vi "Gui.vi"(0 "reference in":refnum<class "RemoteControl.lvclass">, 5 "error in (no error)":errorcluster) -> (14 "reference out":refnum<class "RemoteControl.lvclass">, 19 "error out":errorcluster)   [LabVIEW 2012, in "RemoteControl.lvclass"]
uses:
  RemoteControl.lvclass
  Command_class/Command.lvclass
panel:
  in  "UndoLastCommand":bool
  in  "Slot2_Off":bool
  in  "Slot2_On":bool
  in  "Slot1_Off":bool
  in  "Slot1_On":bool
  in  "Slot0_Off":bool
  in  "Slot0_On":bool
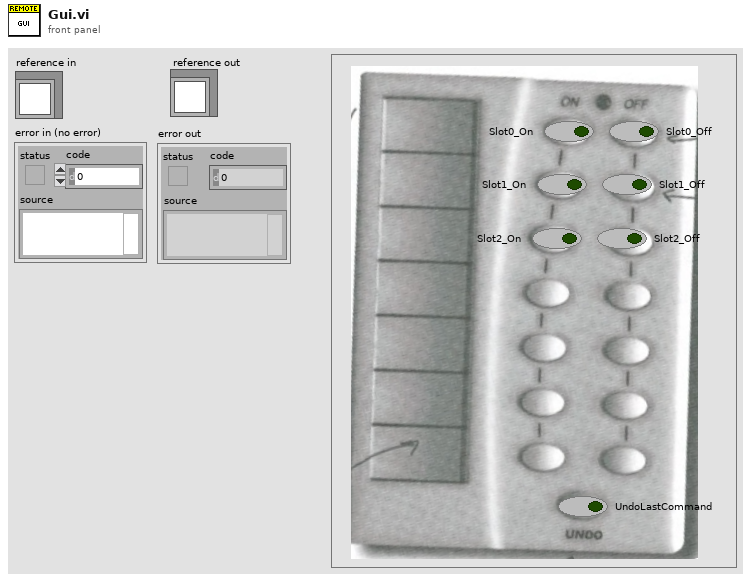
[diagram p1: front panel]
types:
  T1 = cluster{"Event":refnum<event-registration>, "Command":string, "Data":variant, "UndoCommand":refnum<class "Command.lvclass">}
  T2 = typedef "RemoteControl.lvclass/ObjectAttributes.ctl" = cluster{"OnCommands":refnum<class "Command.lvclass">[], "OffCommands":refnum<class "Command.lvclass">[], "UndoCommand":refnum<class "Command.lvclass">}
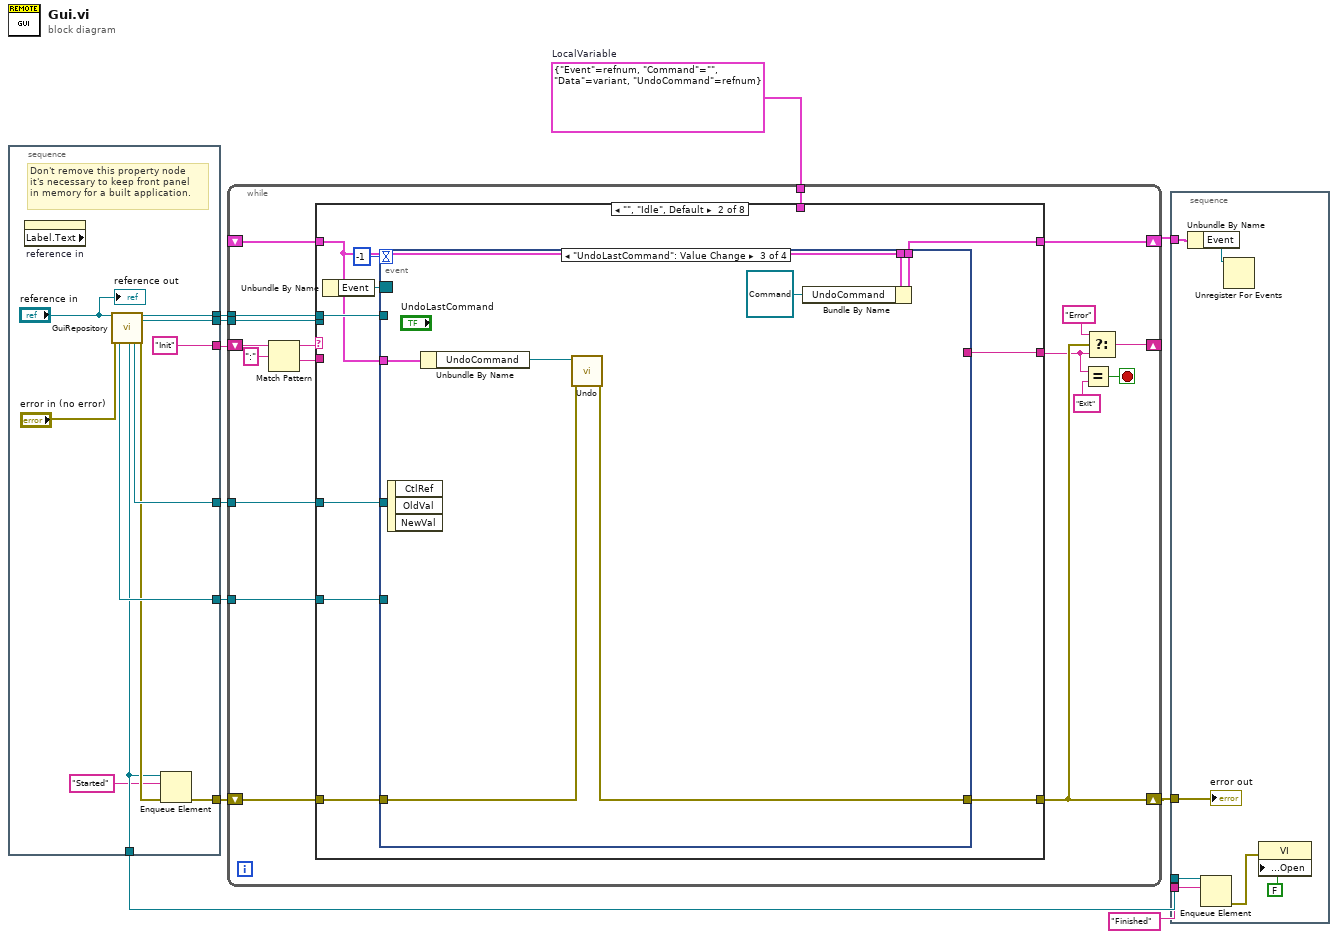
[diagram p0: block diagram]
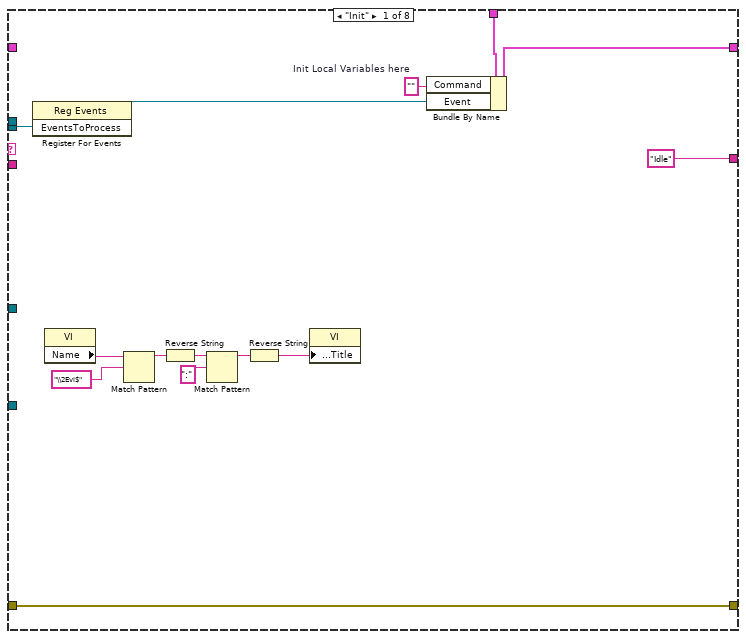
[diagram p2: hidden frame]
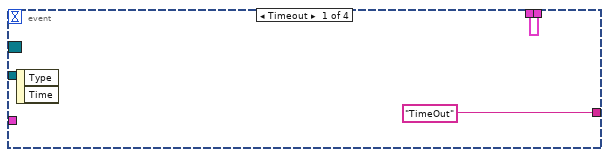
[diagram p3: hidden frame]
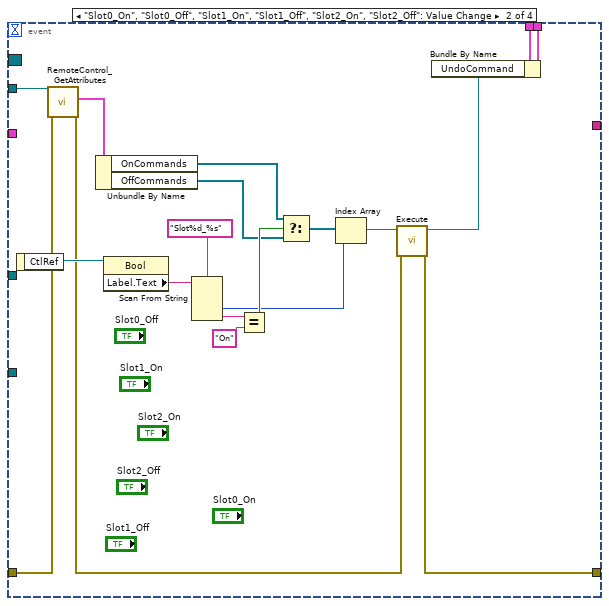
[diagram p4: hidden frame]
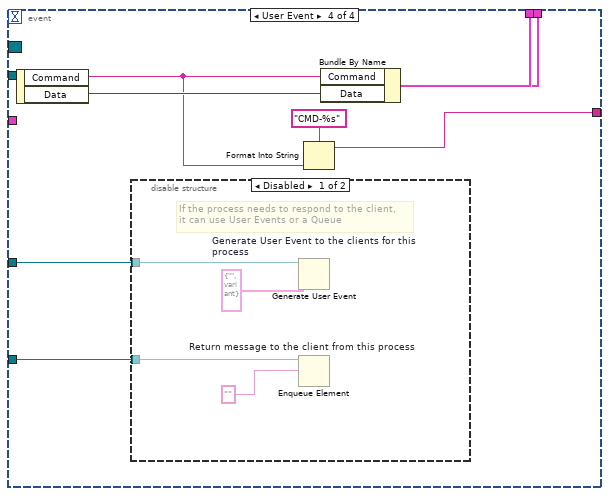
[diagram p5: hidden frame]
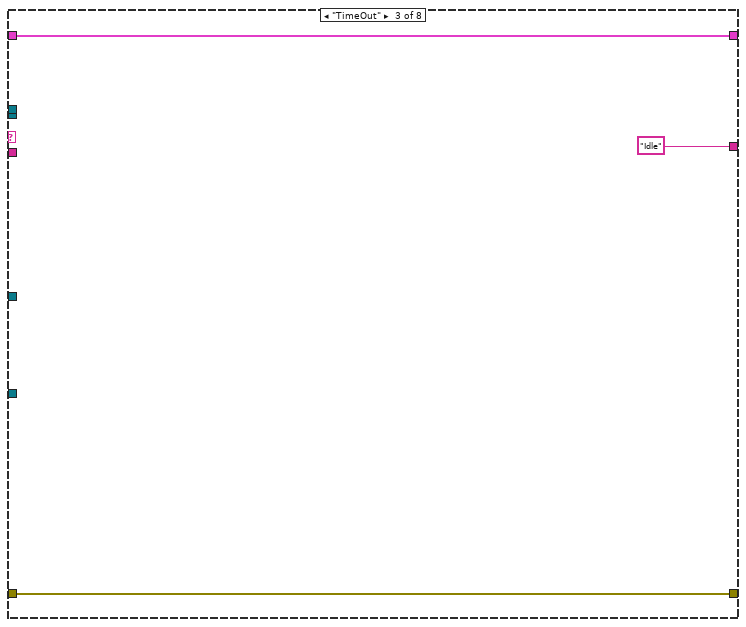
[diagram p7: hidden frame]
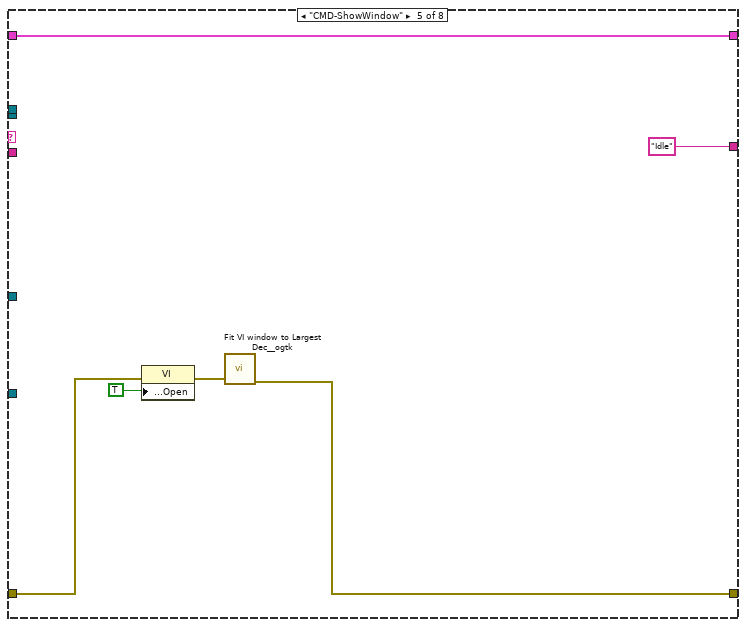
[diagram p9: hidden frame]
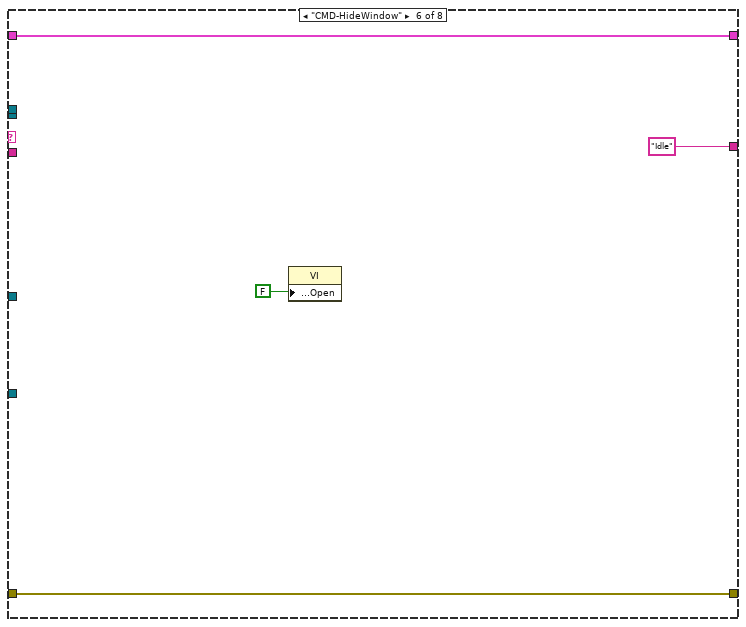
[diagram p10: hidden frame]
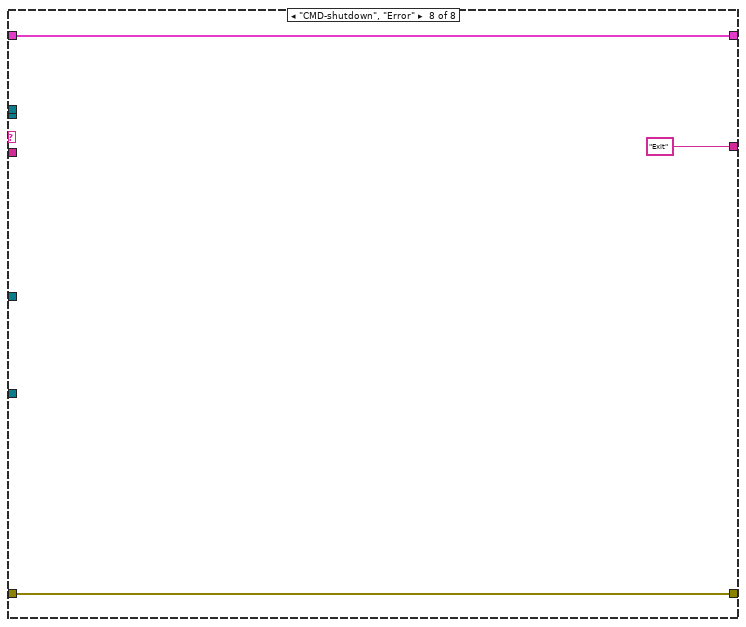
[diagram p12: hidden frame]
diagram:
  w5 = T1 {"Event"=refnum, "Command"="", "Data"=variant, "UndoCommand"=refnum}  # LocalVariable
  n1 = stacked-sequence {
    tunnel: [w13] -> w11
    tunnel: [w22] -> w9
    tunnel: [w19] -> w8
    tunnel: [w14] -> w7
    tunnel: ["Init"] -> w6
    tunnel: [w17] -> w3
    tunnel: [w16] -> w2
    frame #0 {
      # "Don't remove this property node\nit's necessary to keep front panel\nin memory for a built application."
      n2 = property on="reference in" class="LVClassControl (strict)" props=["Label", "Text"]() -> ()  [unwired: 2 in, 3 out]
      n3 = call "GuiRepository.vi"("reference in"="reference in", "error in (no error)"="error in (no error)") -> ("QueueFromProcess"=w16:refnum<queue>, "ProcessSyncQueue"=w14:refnum<queue>, "EventFromProcess"=w17:refnum<user-event>, "reference out"=w22:refnum<class "RemoteControl.lvclass">, "EventsToProcess"=w19:refnum<user-event>, "error out"=w15:errorcluster)  [unwired: 10 in, 2 out]
      n4 = Enqueue Element(queue=w14, element="Started", error in (no error)=w15) -> (error out=w13:errorcluster)  [unwired: 1 in, 2 out]
      "reference out" <- "reference in"
    }
  }
  n5 = while {
    shift-right: [w33] -> w10
    shift-left: w11 -> [w38]
    tunnel: w9 -> [w39]
    tunnel: w8 -> [w40]
    shift-right: [w31] -> _
    shift-left: w6 -> [w36]
    shift-right: [w27] -> w4
    shift-left: _ -> [w26]
    tunnel: w5 -> [w25]
    tunnel: w3 -> [w24]
    tunnel: w2 -> [w23]
    stop <- w28 stop-if-true
    n6 = Match Pattern(string=w36, regular expression=":") -> (before substring=w35:string, after substring=w34:string)  [unwired: 1 in, 2 out]
    n7 = case shown="\"\", \"Idle\", Default" w35 {
      tunnel: w38 -> [w52 w57 w107 w109 w111 w119 w121 w124]
      tunnel: [w52 w56 w107 w109 w110 w119 w121 w124] -> w33
      tunnel: w40 -> [w50 _ _ _ _ _ _ _]
      tunnel: w39 -> [_ w58 _ _ _ _ _ _]
      tunnel: w34 -> [_ _ _ _ _ _ _ _]
      tunnel: ["Idle" ("t") w64 "Idle" ("t") _ "Idle" ("t") "Idle" ("t") _ "Exit" ("y")] -> w30
      tunnel: [w54 w63 w105 w108 w115 w118 w120 w122] -> w27
      tunnel: w26 -> [_ w55 w105 w108 w115 w118 w120 w122]
      tunnel: w25 -> [w48 _ _ _ _ _ _ _]
      tunnel: w24 -> [_ w60 _ _ _ _ _ _]
      tunnel: w23 -> [_ w59 _ _ _ _ _ _]
      frame "Init" {
        w53 = ""  # Init Local Variables here
        n8 = register-events(w50) -> (reference out=w49:refnum<event-registration>)  [unwired: 2 in, 1 out]
        n9 = property class="VI"() -> ("Name"=w47:string)  [unwired: 2 in, 2 out]
        n10 = Match Pattern(string=w47, regular expression="\\2Evi$") -> (before substring=w45:string)  [unwired: 1 in, 3 out]
        n11 = Reverse String(1:w45) -> (0:w44:string)
        n12 = Match Pattern(string=w44, regular expression=":") -> (before substring=w42:string)  [unwired: 1 in, 3 out]
        n13 = Reverse String(1:w42) -> (0:w41:string)
        n14 = property class="VI"("Front Panel.Title"=w41) -> ()  [unwired: 2 in, 2 out]
        n15 = Bundle By Name(cluster=w48, "Command"=w53, "Event"=w49) -> (w54:T1)
      }
      frame "", "Idle", Default {
        n16 = Unbundle By Name(w55) -> ("Event"=w62:refnum<event-registration>)
        n17 = event shown="[2] \"UndoLastCommand\": Value Change" {
          selector: w62 -> [_ _ _ _]
          dyn-events: _ -> [_ _ _ _]
          timeout: -1 -> [_ _ _ _]
          tunnel: ["TimeOut" ("t") _ _ w96] -> w64
          tunnel: w55 -> [w65 w85 w91 w100]
          tunnel: [w65 w68 w90 w99] -> w63
          tunnel: w60 -> [_ _ _ w94]
          tunnel: w59 -> [_ _ _ w93]
          tunnel: w58 -> [_ w84 _ _]
          tunnel: w57 -> [_ w83 w87 _]
          tunnel: [_ w69 w86 _] -> w56
          tunnel: w55 -> [_ _ w92 _]
          event Timeout {
            n18 = event-data() -> ()  [unwired: 1 in, 2 out]
          }
          event "Slot0_On", "Slot0_Off", "Slot1_On", "Slot1_Off", "Slot2_On", "Slot2_Off": Value Change {
            n19 = event-data() -> ("CtlRef"=w81:refnum<vi>)  [unwired: 1 in]
            n20 = call "RemoteControl_GetAttributes.vi"("error in (no error)"=w83, "reference in"=w84) -> ("error out"=w70:errorcluster, "Data"=w82:T2)  [unwired: 6 in, 2 out]
            n21 = Unbundle By Name(w82) -> ("OnCommands"=w75:refnum<class "Command.lvclass">[], "OffCommands"=w74:refnum<class "Command.lvclass">[])
            n22 = property class="Bool"(reference=w81) -> ("Label.Text"=w80:string)  [unwired: 1 in, 2 out]
            n23 = Scan From String(format string="Slot%d_%s", input string=w80) -> (output 1=w72:i32, output 2=w78:string)  [unwired: 4 in, 3 out]
            n24 = Equal?(x=w78, y="On") -> (x = y?=w76:bool)
            n25 = Select(t=w75, s=w76, f=w74) -> (s? t:f=w73:refnum<class "Command.lvclass">[])
            n26 = Index Array(array=w73, index=w72) -> (element=w71:refnum<class "Command.lvclass">)
            n27 = call-dynamic "Execute.vi"("error in (no error)"=w70, "reference in"=w71) -> ("error out"=w69:errorcluster, "reference out"=w67:refnum<class "Command.lvclass">)  [unwired: 8 in]
            n28 = Bundle By Name(cluster=w85, "UndoCommand"=w67) -> (w68:T1)
          }
          event "UndoLastCommand": Value Change {
            n29 = event-data() -> ()  [unwired: 1 in, 3 out]
            n30 = Unbundle By Name(w92) -> ("UndoCommand"=w88:refnum<class "Command.lvclass">)
            n31 = call-dynamic "Undo.vi"("error in (no error)"=w87, "reference in"=w88) -> ("error out"=w86:errorcluster)  [unwired: 8 in, 1 out]
            n32 = Bundle By Name(cluster=w91, "UndoCommand"=refnum<class "Command.lvclass"> refnum) -> (w90:T1)
          }
          event User Event {
            n33 = event-data() -> ("Command"=w95:string, "Data"=w98:variant)  [unwired: 1 in]
            n34 = disable-structure shown="Disabled" {
              disable-tunnel: w94 -> [w104 _]
              disable-tunnel: w93 -> [w103 _]
              frame Disabled {
                # "If the process needs to respond to the client,\nit can use User Events or a Queue"
                n35 = Generate User Event "Generate User Event to the clients for this process"(user event=w104, event data cluster=cluster{"Command":string, "Data":variant} {"Command"="", "Data"=variant} ("event data")) -> ()  [unwired: 1 in, 2 out]
                n36 = Enqueue Element "Return message to the client from this process"(queue=w103, element="") -> ()  [unwired: 2 in, 3 out]
              }
              frame Enabled {
              }
            }
            n37 = Format Into String(format string="CMD-%s", w95) -> (resulting string=w96:string)  [unwired: 2 in, 1 out]
            n38 = Bundle By Name(cluster=w100, "Command"=w95, "Data"=w98) -> (w99:T1)
          }
        }
      }
      frame "TimeOut" {
      }
      frame "---- COMMANDS START----" {
      }
      frame "CMD-ShowWindow" {
        n39 = property class="VI"(error in=w111, "Front Panel.Open"=TRUE ("Front Panel Window:Open")) -> (error out=w112:errorcluster)  [unwired: 1 in, 1 out]
        n40 = call <userlib>:"Fit VI window to Largest Dec__ogtk.vi"("error in (no error)"=w112) -> ("error out"=w110:errorcluster)  [unwired: 5 in, 1 out]
      }
      frame "CMD-HideWindow" {
        n41 = property class="VI"("Front Panel.Open"=FALSE ("Front Panel Window:Open")) -> ()  [unwired: 2 in, 2 out]
      }
      frame "----- COMMANDS END ----" {
      }
      frame "CMD-shutdown", "Error" {
      }
    }
    n42 = Equal?(x=w30, y="Exit") -> (x = y?=w28:bool)
    n43 = Select(t="Error", s=w33, f=w30) -> (s? t:f=w31:string)
  }
  n44 = stacked-sequence {
    tunnel: w10 -> [w131]
    tunnel: w7 -> [w127]
    tunnel: w4 -> [w130]
    tunnel: "Finished" ("element") -> [w125]
    frame #0 {
      n45 = Unbundle By Name(w130) -> ("Event"=w129:refnum<event-registration>)
      n46 = Enqueue Element(queue=w127, element=w125) -> (error out=w126:errorcluster)  [unwired: 2 in, 2 out]
      n47 = Unregister For Events(event registration refnum=w129) -> ()  [unwired: 1 in, 1 out]
      n48 = property class="VI"(error in=w126, "Front Panel.Open"=FALSE ("Front Panel Window:Open")) -> ()  [unwired: 1 in, 2 out]
      "error out" <- w131
    }
  }
